vi "EEI EXP6.vi"() -> ()   [LabVIEW 2020]
panel:
  out "d>=0 case":bool
  out "d":dbl
  out "current time":timestamp
  out "Y":dbl
  in  "y":dbl
  in  "x":dbl
  out "n":dbl
  out "m":dbl
  in  "c":dbl
  in  "b":dbl
  in  "a":dbl
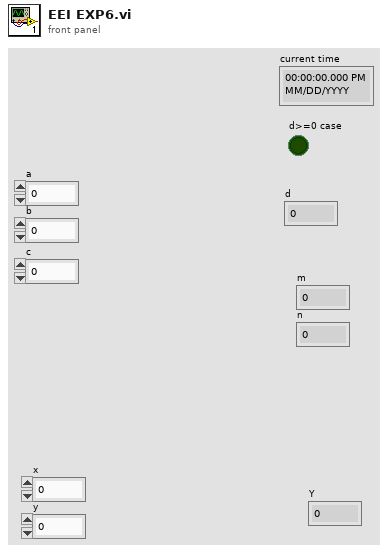
[diagram p1: front panel]
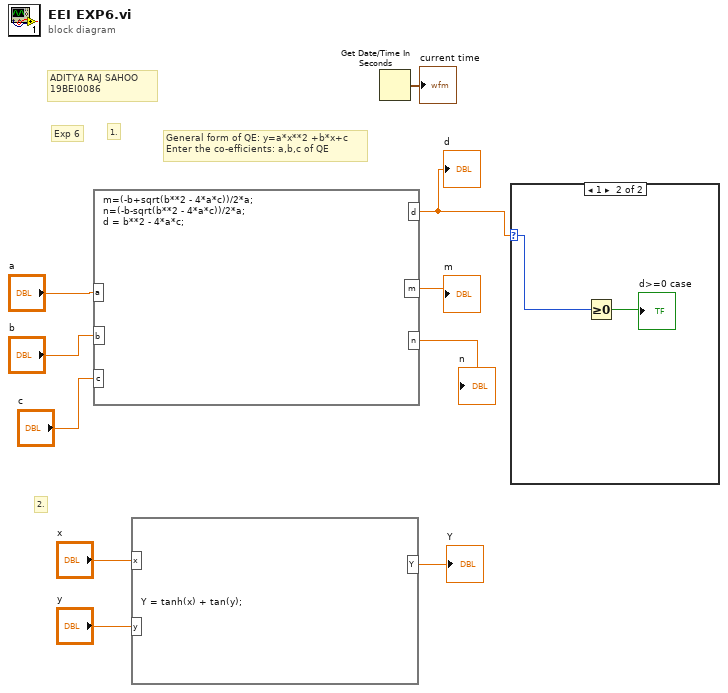
[diagram p0: block diagram]
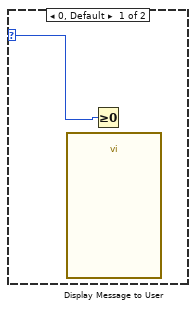
[diagram p2: hidden frame]
diagram:
  # "2."
  # "General form of QE: y=a*x**2 +b*x+c \nEnter the co-efficients: a,b,c of QE"
  # "1."
  # "Exp 6"
  # "ADITYA RAJ SAHOO\n19BEI0086"
  n1 = formula code="m=(-b+sqrt(b**2 - 4*a*c))/2*a;\nn=(-b-sqrt(b**2 - 4*a*c))/2*a;\nd = b**2 - 4*a*c;"("a"="a", "b"="b", "c"="c") -> ("m"=→"m":dbl, "n"=→"n":dbl, "d"=w1:dbl)
  "d" <- w1
  n2 = formula code="Y = tanh(x) + tan(y);"("x"="x", "y"="y") -> ("Y"=→"Y":dbl)
  n3 = Get Date/Time In Seconds() -> (seconds since 1Jan1904=→"current time":timestamp)
  n4 = case shown="1" w1 {
    selector: w1 -> [w11 w13]
    frame 0, Default {
      n5 = call "Display Message to User"() -> ()  [unwired: 10 in, 2 out]
      n6 = Greater Or Equal To 0?(x=w11) -> ()  [unwired: 1 out]
    }
    frame 1 {
      n7 = Greater Or Equal To 0?(x=w13) -> (x >= 0?=→"d>=0 case":bool)
    }
  }
